vi "主程序-复材超声C扫缺陷分析评定软件.vi"() -> ()   [LabVIEW 2018]
doc: "使用该模板构建用户界面事件处理设计模式。将模板应用于对话框及其它用户界面。用户也可创建并执行VI可按照与用户界面事件相同方式处理的用户定义事件。"
uses:
  <vilib>/Utility/NIReport.llb/Report Type.ctl
  <vilib>/addons/_office/_exclsub.llb/font.ctl
  <vilib>/Utility/NIReport.llb/HTML Report Image Alignment.ctl
  <vilib>/Utility/NIReport.llb/Append Report Text (str wrap).vi
  <vilib>/Utility/NIReport.llb/Append Image to Report (path wrap).vi
  <vilib>/addons/_office/word.llb/Word Easy Table (str).vi
  <vilib>/Utility/NIReport.llb/NI_report.lvclass
  <vilib>/Utility/NIReport.llb/Word/NI_Word.lvclass
  <vilib>/addons/_office/NI_ReportGenerationToolkit.lvlib
  <vilib>/Utility/NIReport.llb/NI_ReportGenerationCore.lvlib
  <vilib>/vision/NI_Vision_Development_Module.lvlib
panel:
  out "报告模式":string
  in  "删除标注":bool caption="定量分析"
  out "输入的灰度阈值":dbl caption="值"
  out "反射图原始路径":path
  out "穿透图原始路径":path
  out "ROImask":T1(plugin-control)
  out "模式选择":u16(ring) items=["只读穿透图", "穿透图和反射图结合"]
  out "添加的路径":path
  out "连接的字符串 2":string
  out "临界面积百分比值":dbl
  out "临界Z值":i32
  out "标注后的图片路径":path
  out "弥散类检测结果合并":string[][](table)
  out "分层类检测结果合并":string[][](table)
  out "弥散类检测结果":string[][](table)
  out "分层类检测结果":string[][](table)
  out "部位信息":string[](array[string])=["", "34.500000", "32.500000", "1121", "34", "54.955926", "分层类", "不合格", ""]
  out "连接的字符串":string
  in  "完成标注":bool caption="定量分析"
  out "框数":dbl
  out "自定义字体":T2={"Desired Font (Application)"=enum."Application Font", "[User-specified Font]"={"Font Name"="", "Size"=12, "Strikeout?"=FALSE, "Italic?"=FALSE, "Underline?"=FALSE, "Outline?"=FALSE, "Shadow?"=FALSE, "Bold?"=FALSE, "Rotation Angle"=0.0}, "Horizontal Alignment"=0, "Vertical Alignment"=0} {"Horizontal Alignment" items=["Left", "Center", "Right"]; "Vertical Alignment" items=["Bottom", "Top", "Baseline"]}
  out "框组":T3(array[cluster])
  out "质量等级":string
  out "灰度阈值":dbl
  in  "stop":bool caption="停止"
  in  "导入图像":bool caption="导入图片"
  in  "开始标注":bool caption="定量分析"
  in  "查看评定结果":bool caption="辅助定性分析"
  in  "生成报告":bool caption="生成原始记录"
  in  "控件":enum32{"穿透图", "反射图"}(tab)
  out "穿透图":T1(plugin-control)
  out "反射图":T1(plugin-control)
  out "产品规格":cluster{"产品长度（周长）（mm）":dbl, "产品宽度（母线长）（mm）":dbl}
  out "图像分辨率":T4
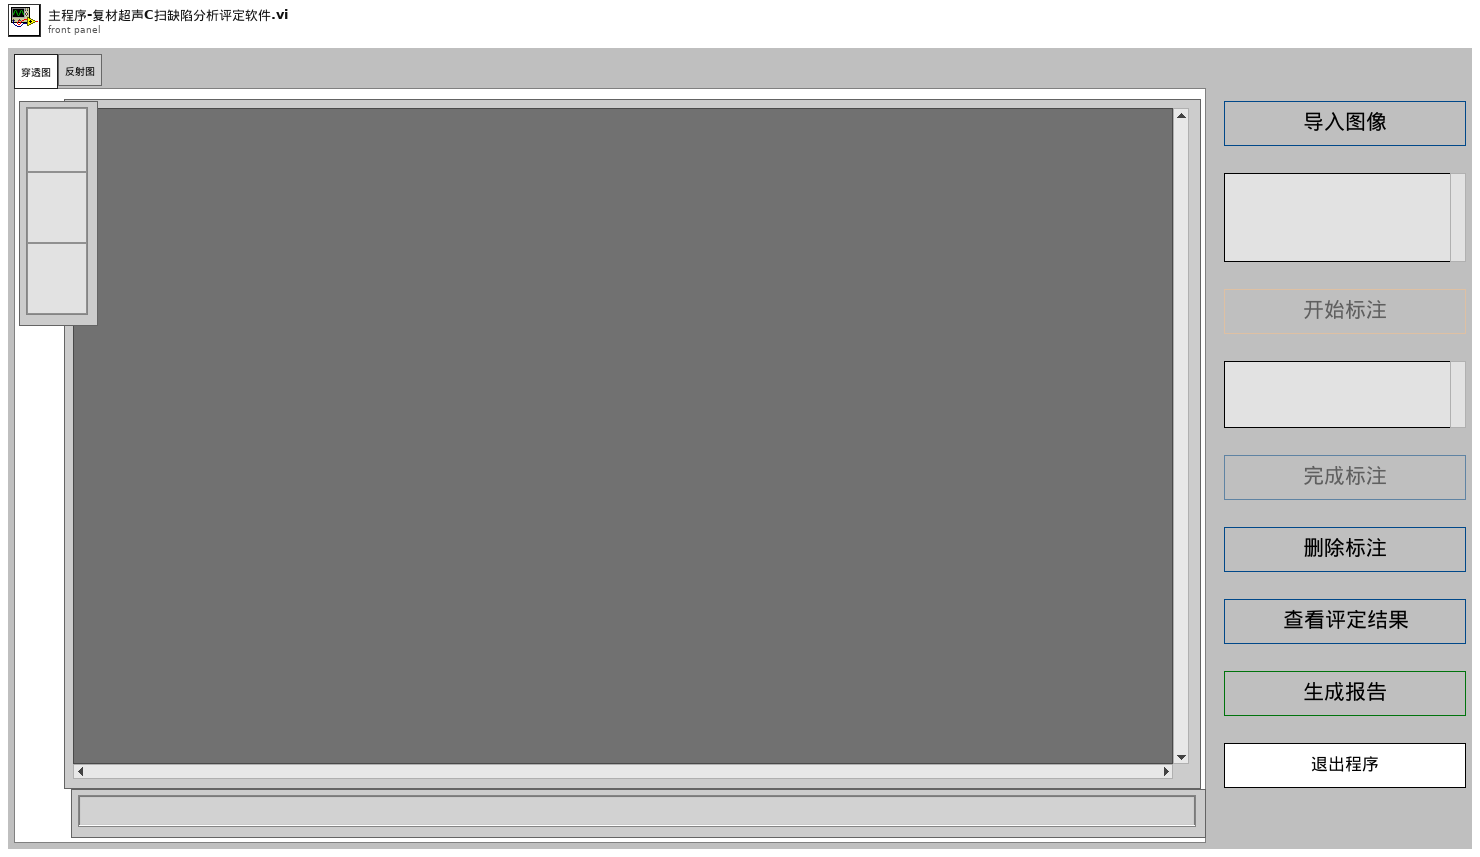
[diagram p1: front panel]
types:
  T1 = typedef "IMAQ Image.ctl" = refnum<image>
  T2 = cluster{"Desired Font (Application)":enum16{"User-specified Font", "Application Font", "System Font", "Dialog Font"}, "[User-specified Font]":cluster{"Font Name":string, "Size":i16, "Strikeout?":bool, "Italic?":bool, "Underline?":bool, "Outline?":bool, "Shadow?":bool, "Bold?":bool, "Rotation Angle":dbl}, "Horizontal Alignment":i16, "Vertical Alignment":i16}
  T3 = cluster{"Global Rectangle":i32[], "Contours":cluster{"Contour Type":u32, "ROI Type":u32, "Points":i32[]}[]}[]
  T4 = cluster{"图像X向分辨率（mm/像素）":dbl, "图像Y向分辨率（mm/像素）":dbl}
  T5 = enum8{"Enabled", "Disabled", "Disabled and Grayed Out"}
  T6 = cluster{"Global Rectangle":i32[], "Contours":cluster{"Contour Type":u32, "ROI Type":u32, "Points":i32[]}[]}
  T7 = cluster{"Zoom Tool":bool, "Selection Tool":bool, "Pan Tool":bool, "Point Tool":bool, "Line Tool":bool, "Rectangle Tool":bool, "Rotated Rectangle Tool":bool, "Polyline Tool":bool, "Polygon Tool":bool, "Freehand Tool":bool, "Closed Freehand Tool":bool, "Ellipse Tool":bool, "Annulus Tool":bool}
  T8 = enum16{"maximized", "minimized", "normal", "no change"}
  T9 = typedef "NI_ReportGenerationCore.lvlib/Report Type.ctl" = enum16{"HTML", "Word", "Excel"}
  T10 = cluster{"position (excel)":cluster{"row":i32, "column":i32}, "name (excel)":string, "bookmark (word)":string}
  T11 = typedef "NI_ReportGenerationCore.lvlib/HTML Report Image Alignment.ctl" = enum16{"(default)", "LEFT", "RIGHT", "TOP", "TEXTTOP", "MIDDLE", "ABSMIDDLE", "BASELINE", "BOTTOM", "ABSBOTTOM"}
  T12 = cluster{"position (Excel)":cluster{"row":i32, "column":i32}, "name (Excel)":string, "bookmark (Word)":string}
  T13 = typedef "NI_ReportGenerationToolkit.lvlib/font.ctl" = cluster{"font name":string, "font size":dbl, "bold":u16, "italic":u16, "underline":u16, "strike through":u16, "font color":u32}
  T14 = typedef "Image Type" = u32
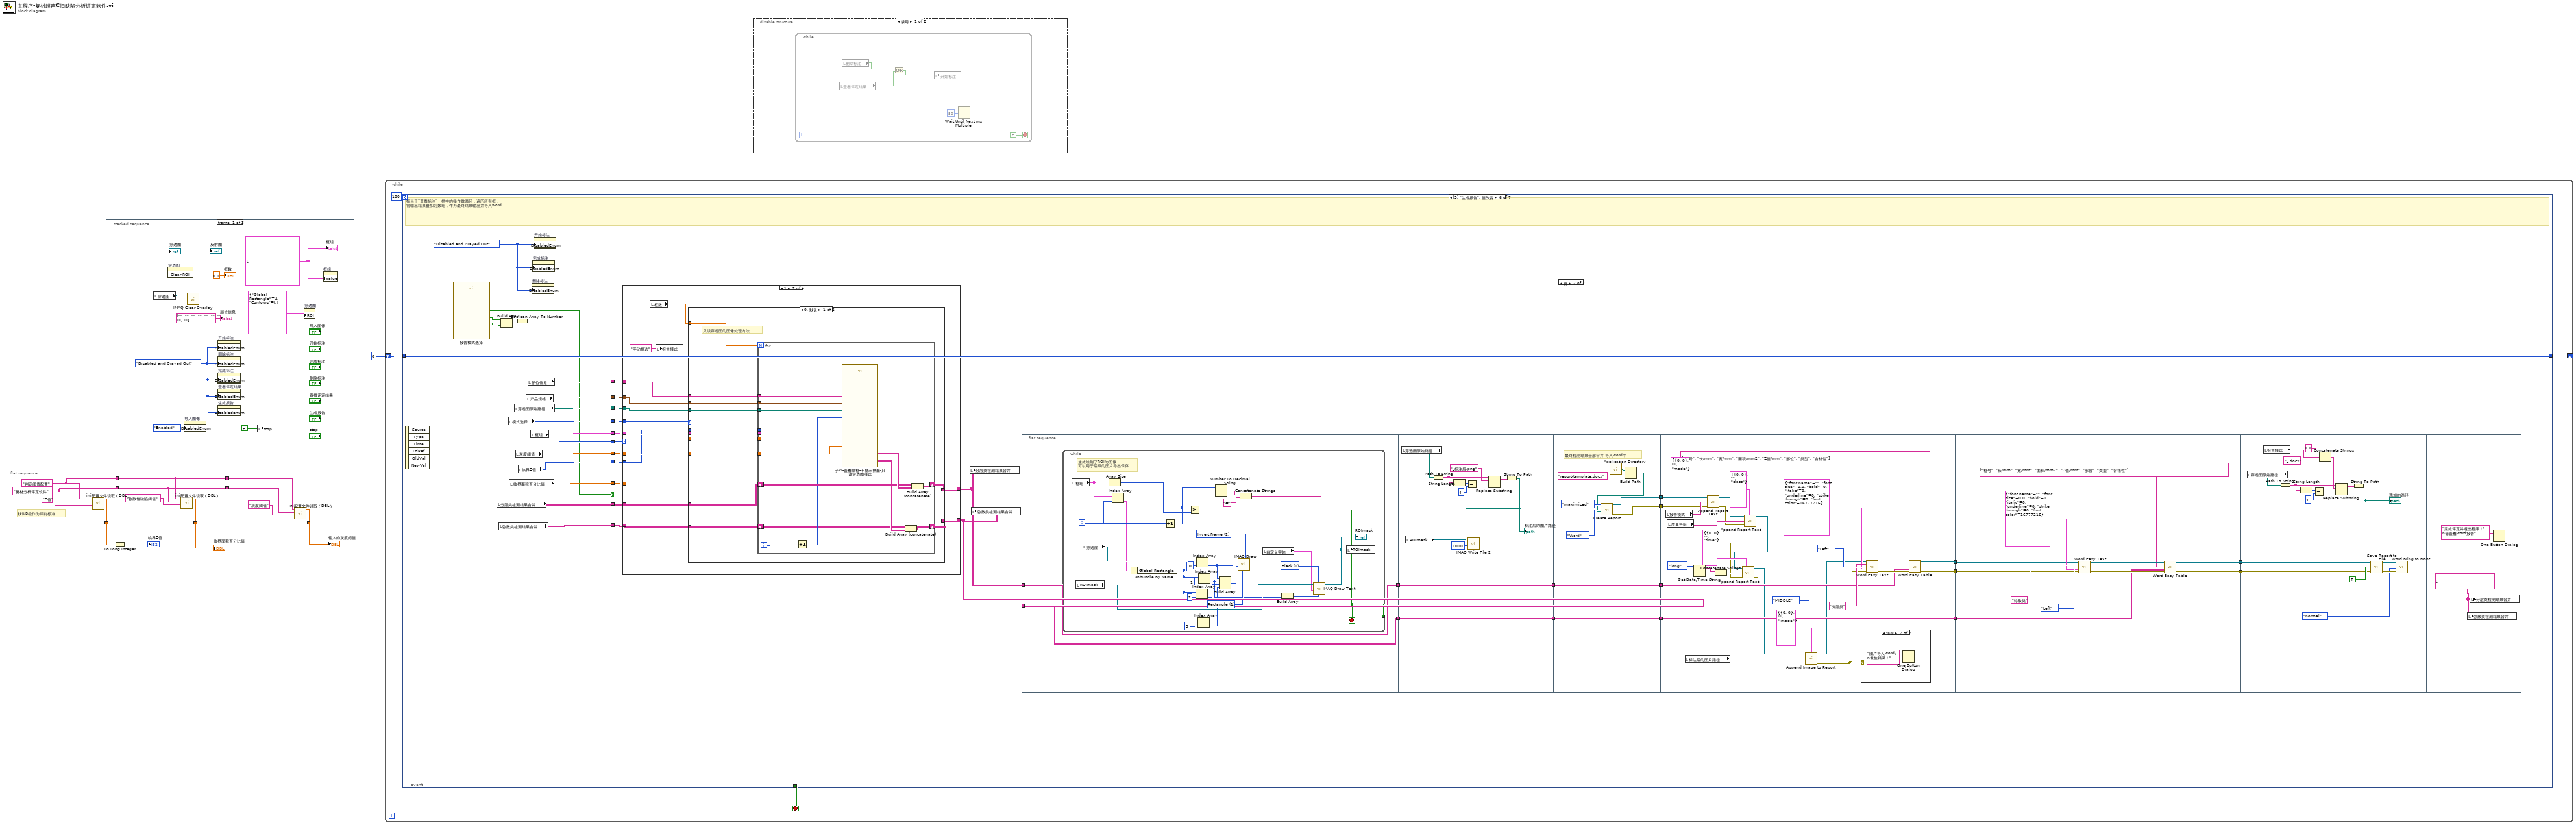
[diagram p0: block diagram]
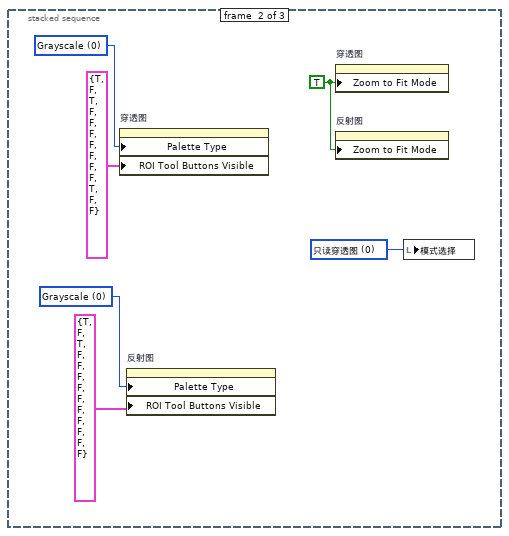
[diagram p2: hidden frame]
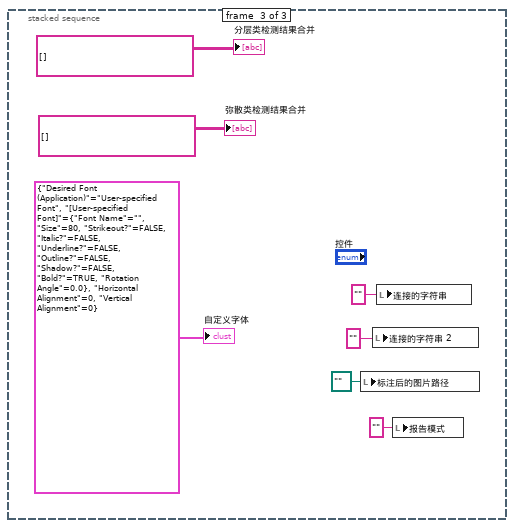
[diagram p3: hidden frame]
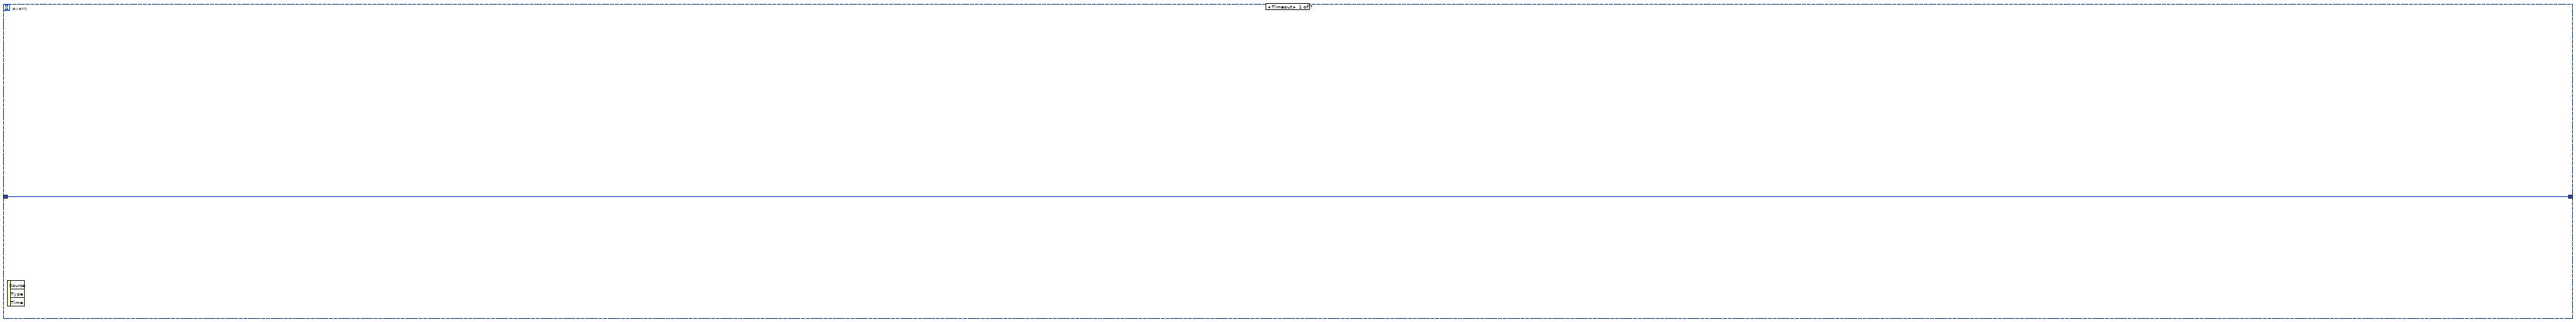
[diagram p5: hidden frame]
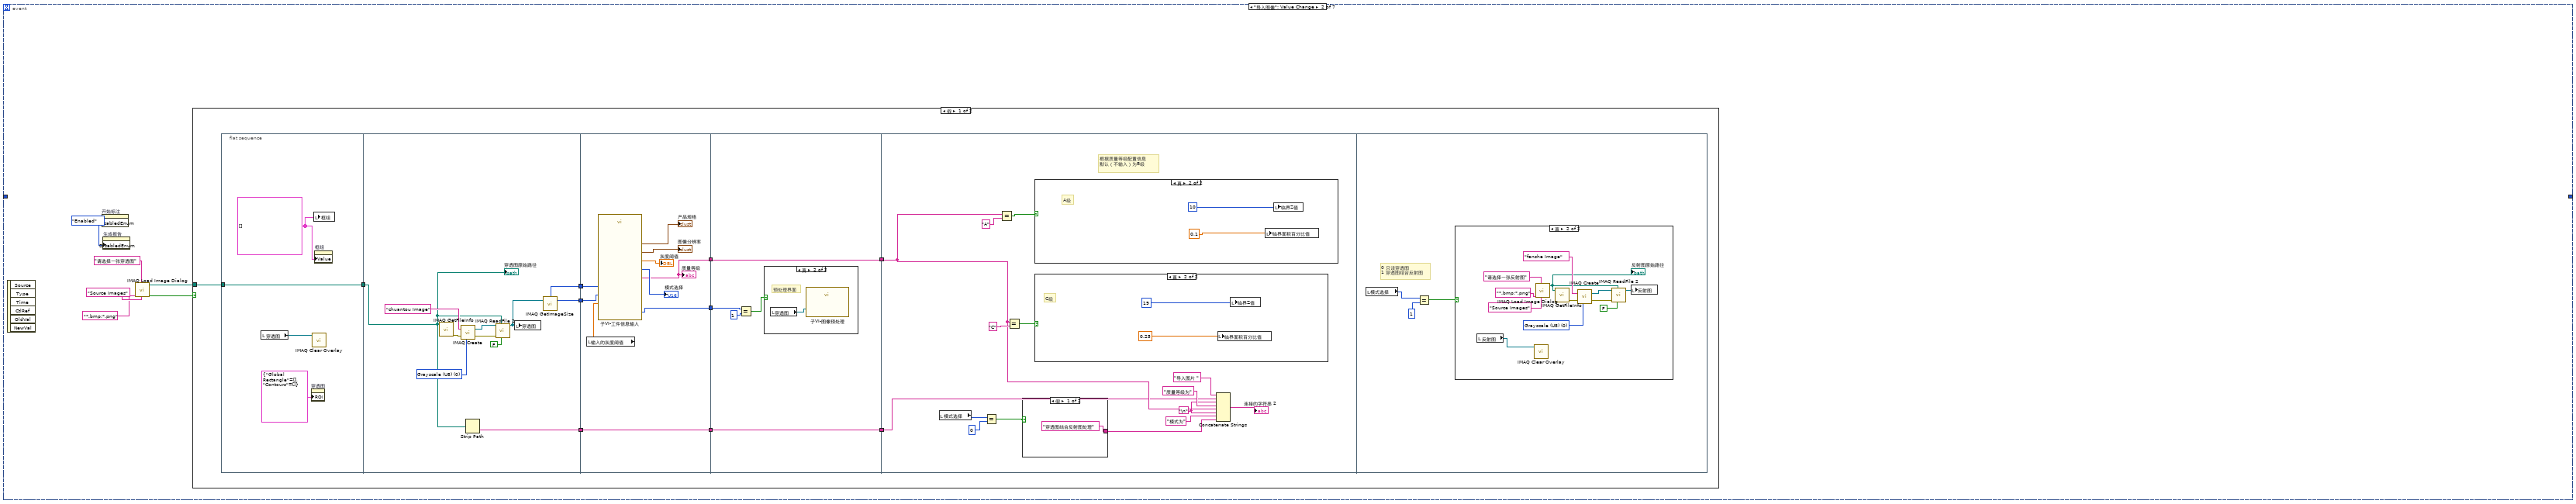
[diagram p6: hidden frame]
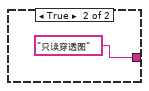
[diagram p8: hidden frame]
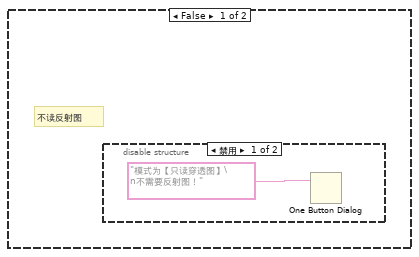
[diagram p11: hidden frame]
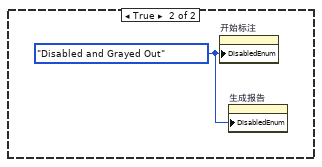
[diagram p13: hidden frame]
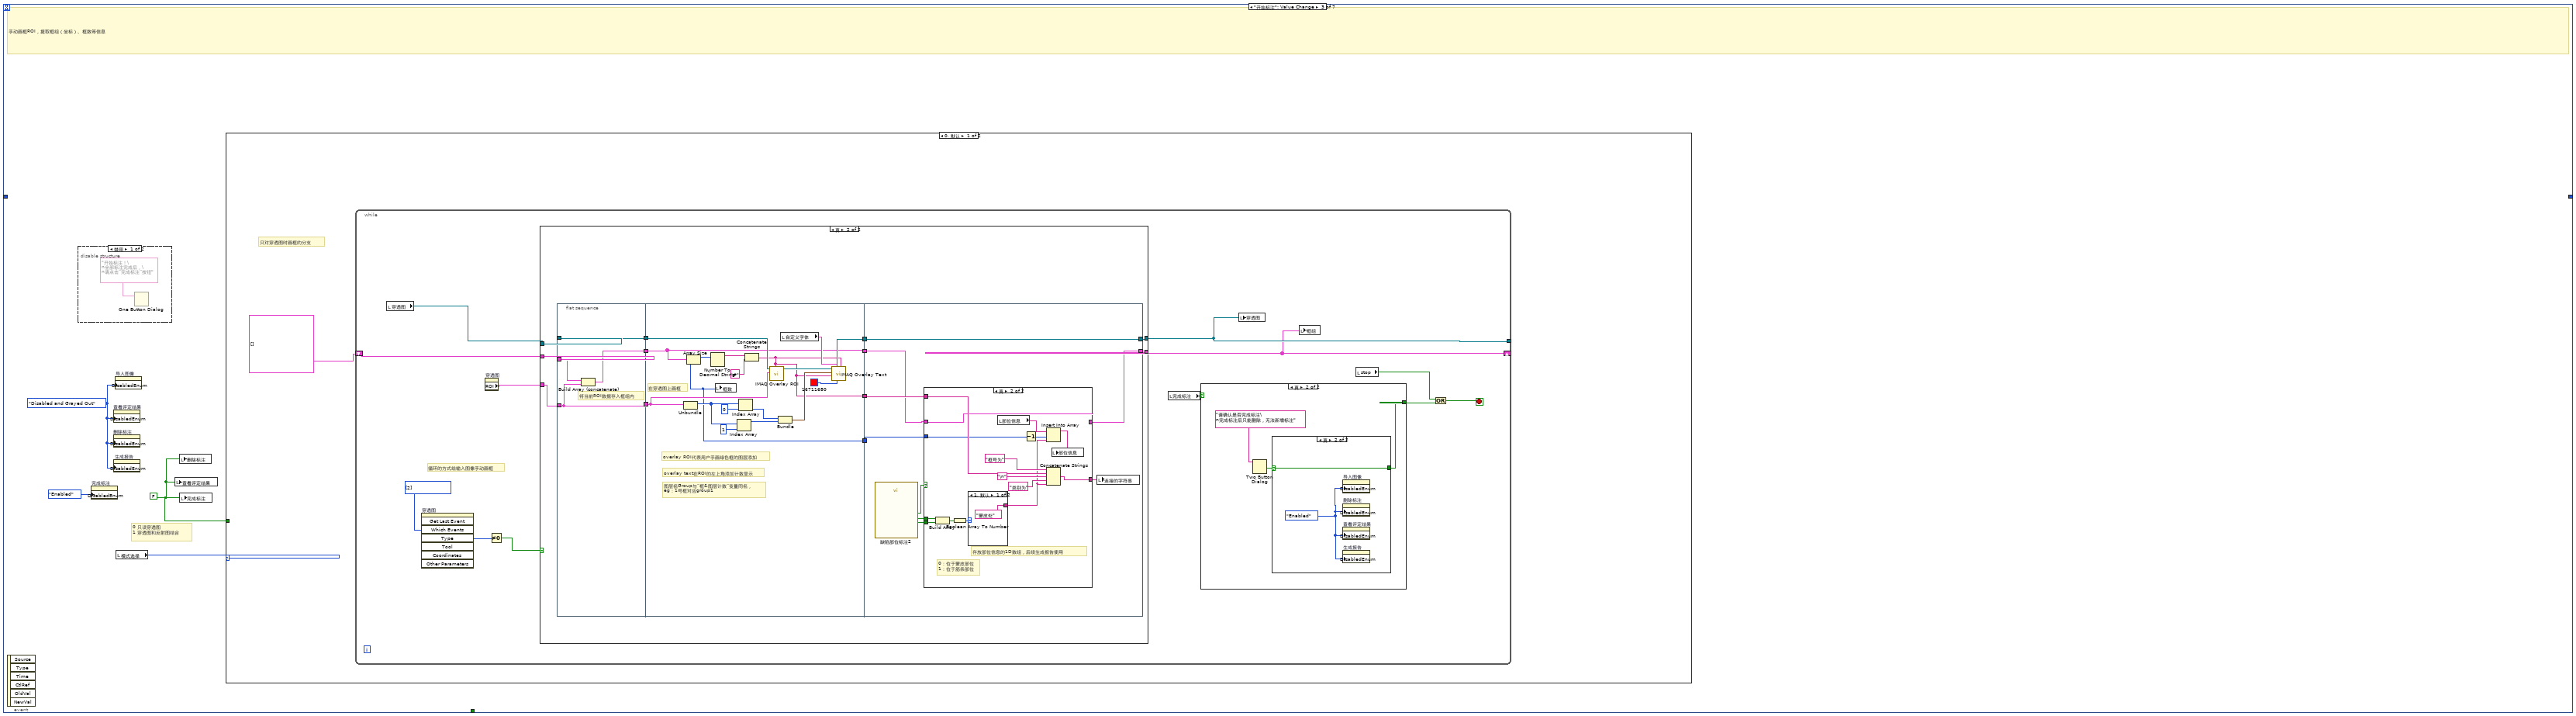
[diagram p14: hidden frame]
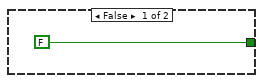
[diagram p16: hidden frame]
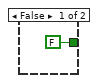
[diagram p17: hidden frame]
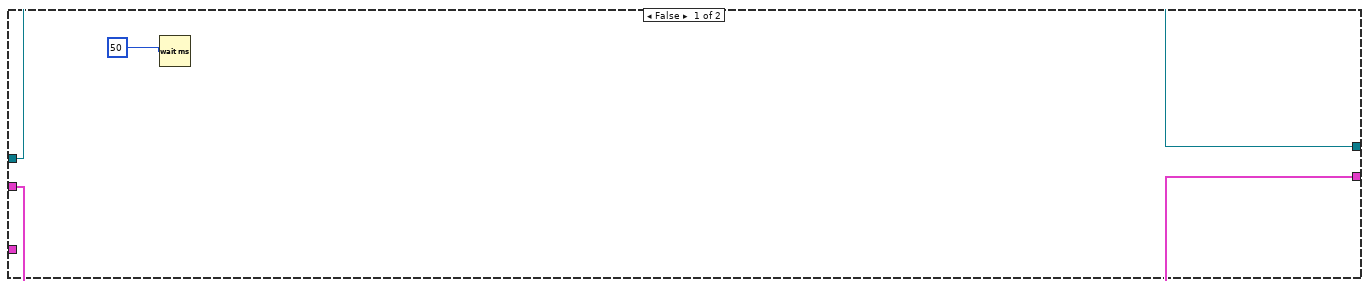
[diagram p18: hidden frame]
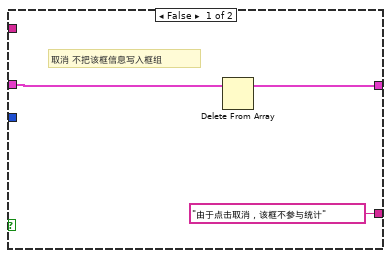
[diagram p19: hidden frame]
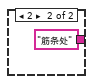
[diagram p20: hidden frame]
diagram:
  n1 = flat-sequence {
    tunnel: [w12] -> w8
    tunnel: [w11] -> w7
    tunnel: [w10] -> w2
    tunnel: w8 -> [w15]
    tunnel: w7 -> [w16]
    tunnel: [w16] -> w6
    tunnel: [w15] -> w5
    tunnel: [w14] -> w3
    tunnel: w6 -> [w20]
    tunnel: w5 -> [w19]
    tunnel: [w18] -> w4
    frame #0 {
      w11 = "复材分析评定软件" ("section")
      w12 = "判定阈值配置" ("文件名称")
      # "默认B级作为评判标准"
      n2 = call "ini配置文件读取（DBL）.vi"("key"="Z值", "section"=w11, "文件名称"=w12) -> ("value"=w10:dbl)  [unwired: 8 in]
    }
    frame #1 {
      n3 = call "ini配置文件读取（DBL）.vi"("key"="弥散性缺陷阈值", "section"=w16, "文件名称"=w15) -> ("value"=w14:dbl)  [unwired: 8 in]
    }
    frame #2 {
      n4 = call "ini配置文件读取（DBL）.vi"("key"="灰度阈值", "section"=w20, "文件名称"=w19) -> ("value"=w18:dbl)  [unwired: 8 in]
    }
  }
  n5 = stacked-sequence {
    frame #0 {
      w27 = T3 [] ("框组")
      w23 = T5."Disabled and Grayed Out" ("禁用")
      n6 = local read "穿透图"() -> (w25:T1)
      n7 = invoke on="穿透图" class="ImageControl" method="Clear ROI"() -> ()  [unwired: 3 in, 3 out]
      n8 = property on="导入图像" class="Bool"("DisabledEnum"=T5."Enabled" ("禁用")) -> ()  [unwired: 2 in, 2 out]
      n9 = call "IMAQ Clear Overlay"("Image"=w25) -> ()  [unwired: 9 in, 2 out]
      n10 = property on="开始标注" class="Bool"("DisabledEnum"=w23) -> ()  [unwired: 2 in, 2 out]
      n11 = property on="删除标注" class="Bool (严格)"("DisabledEnum"=w23) -> ()  [unwired: 2 in, 2 out]
      n12 = property on="完成标注" class="Bool (严格)"("DisabledEnum"=w23) -> ()  [unwired: 2 in, 2 out]
      n13 = property on="查看评定结果" class="Bool (严格)"("DisabledEnum"=w23) -> ()  [unwired: 2 in, 2 out]
      n14 = property on="生成报告" class="Bool"("DisabledEnum"=w23) -> ()  [unwired: 2 in, 2 out]
      n15 = local write "stop"(FALSE ("stop")) -> ()
      n16 = property on="穿透图" class="ImageControl"("ROI"=T6 {"Global Rectangle"=[], "Contours"=[]}) -> ()  [unwired: 2 in, 2 out]
      n17 = property on="框组" class="Arr (严格)"("Value"=w27) -> ()  [unwired: 2 in, 2 out]
      "部位信息" <- string[] ["", "", "", "", "", "", "", "", ""] ("部位信息")
      "框组" <- w27
      "框数" <- 0.0 ("框数")
    }
    frame #1 {
      w30 = u16 0 items=["只读穿透图", "穿透图和反射图结合"] ("模式选择")
      w32 = u32 0 items=["Grayscale", "Binary", "Gradient", "Rainbow", "Temperature", "User Defined", "Binary 16 Bit", "Gradient 16 Bit", "Rainbow 16 Bit", "Temperature 16 Bit", "User Defined 16 Bit"] ("Palette:Palette Type")
      w33 = TRUE ("Zoom to Fit Mode")
      w35 = u32 0 items=["Grayscale", "Binary", "Gradient", "Rainbow", "Temperature", "User Defined", "Binary 16 Bit", "Gradient 16 Bit", "Rainbow 16 Bit", "Temperature 16 Bit", "User Defined 16 Bit"] ("Palette:Palette Type")
      n18 = property on="穿透图" class="ImageControl"("Palette Type"=w35, "ROI Tool Buttons Visible"=T7 {"Zoom Tool"=TRUE, "Selection Tool"=FALSE, "Pan Tool"=TRUE, "Point Tool"=FALSE, "Line Tool"=FALSE, "Rectangle Tool"=FALSE, "Rotated Rectangle Tool"=FALSE, "Polyline Tool"=FALSE, "Polygon Tool"=FALSE, "Freehand Tool"=FALSE, "Closed Freehand Tool"=TRUE, "Ellipse Tool"=FALSE, "Annulus Tool"=FALSE} ("ROI Tool Buttons Visible:All Elements")) -> ()  [unwired: 2 in, 2 out]
      n19 = property on="反射图" class="ImageControl"("Palette Type"=w32, "ROI Tool Buttons Visible"=T7 {"Zoom Tool"=TRUE, "Selection Tool"=FALSE, "Pan Tool"=TRUE, "Point Tool"=FALSE, "Line Tool"=FALSE, "Rectangle Tool"=FALSE, "Rotated Rectangle Tool"=FALSE, "Polyline Tool"=FALSE, "Polygon Tool"=FALSE, "Freehand Tool"=FALSE, "Closed Freehand Tool"=FALSE, "Ellipse Tool"=FALSE, "Annulus Tool"=FALSE} ("ROI Tool Buttons Visible:All Elements")) -> ()  [unwired: 2 in, 2 out]
      n20 = property on="穿透图" class="ImageControl"("Zoom to Fit Mode"=w33) -> ()  [unwired: 2 in, 2 out]
      n21 = property on="反射图" class="ImageControl"("Zoom to Fit Mode"=w33) -> ()  [unwired: 2 in, 2 out]
      n22 = local write "模式选择"(w30) -> ()
    }
    frame #2 {
      n23 = local write "标注后的图片路径"(path "" ("标注后的图片路径")) -> ()
      n24 = local write "连接的字符串 2"("" ("连接的字符串 2")) -> ()
      n25 = local write "连接的字符串"("" ("连接的字符串")) -> ()
      n26 = local write "报告模式"("" ("报告模式")) -> ()
      "自定义字体" <- T2 {"Desired Font (Application)"=enum."User-specified Font", "[User-specified Font]"={"Font Name"="", "Size"=80, "Strikeout?"=FALSE, "Italic?"=FALSE, "Underline?"=FALSE, "Outline?"=FALSE, "Shadow?"=FALSE, "Bold?"=TRUE, "Rotation Angle"=0.0}, "Horizontal Alignment"=0, "Vertical Alignment"=0} ("Font, Size & Style")
      "分层类检测结果合并" <- string[][] [] ("弥散类检测结果合并")
      "弥散类检测结果合并" <- string[][] [] ("弥散类检测结果合并")
    }
  }
  n27 = To Long Integer(number=w2) -> (32bit integer=→"临界Z值":i32)
  n28 = while {
    shift-right: [w43] -> _
    shift-left: 0 -> [w44]
    stop <- w46 stop-if-true
    n29 = event shown="[5] \"生成报告\": 值改变" {
      selector: _ -> [_ _ _ _ _ _ _]
      dyn-events: _ -> [_ _ _ _ _ _ _]
      timeout: 100 -> [_ _ _ _ _ _ _]
      tunnel: [_ _ _ _ _ _ w737] -> w46
      tunnel: w44 -> [w47 _ _ _ _ w401 _]
      tunnel: [w47 _ _ _ _ w401 0] -> w43
      event Timeout {
        n30 = event-data() -> ()  [unwired: 1 in, 3 out]
      }
      event "导入图像": Value Change {
        w48 = T5."Enabled" ("禁用")
        n31 = event-data() -> ()  [unwired: 1 in, 6 out]
        n32 = property on="开始标注" class="Bool"("DisabledEnum"=w48) -> ()  [unwired: 2 in, 2 out]
        n33 = property on="生成报告" class="Bool"("DisabledEnum"=w48) -> ()  [unwired: 2 in, 2 out]
        n34 = call "IMAQ Load Image Dialog"("Pattern Label"="Source Images", "Prompt"="请选择一张穿透图" ("prompt"), "Pattern"="*.bmp;*.png") -> ("Cancelled?"=w50:bool, "Path"=w49:path)  [unwired: 6 in, 1 out]
        n35 = case shown="假" w50 {
          tunnel: w49 -> [w60 _]
          frame False {
            n36 = flat-sequence {
              tunnel: w60 -> [w64]
              tunnel: [w64] -> w59
              tunnel: w59 -> [w69]
              tunnel: [w71] -> w58
              tunnel: [w70] -> w57
              tunnel: [w68] -> w56
              tunnel: [w84] -> w63
              tunnel: [w82] -> w62
              tunnel: w58 -> [w81]
              tunnel: w57 -> [w80]
              tunnel: w56 -> [w79]
              tunnel: [w79] -> w55
              tunnel: w63 -> [w93]
              tunnel: [w93] -> w61
              tunnel: w62 -> [w91]
              tunnel: w55 -> [w89]
              tunnel: [w89] -> w54
              tunnel: w61 -> [w102]
              tunnel: w54 -> [w95]
              frame #0 {
                w65 = T3 [] ("框组")
                n37 = local read "穿透图"() -> (w67:T1)
                n38 = property on="穿透图" class="ImageControl"("ROI"=T6 {"Global Rectangle"=[], "Contours"=[]}) -> ()  [unwired: 2 in, 2 out]
                n39 = call "IMAQ Clear Overlay"("Image"=w67) -> ()  [unwired: 9 in, 2 out]
                n40 = local write "框组"(w65) -> ()
                n41 = property on="框组" class="Arr (严格)"("Value"=w65) -> ()  [unwired: 2 in, 2 out]
              }
              frame #1 {
                w73 = T14 0 items=["Grayscale (U8)", "Grayscale (I16)", "Grayscale (SGL)", "Complex (CSG)", "RGB (U32)", "HSL (U32)", "RGB (U64)", "Grayscale (U16)"] ("Image Type")
                n42 = call "IMAQ GetFileInfo"("File Path"=w69) -> ("error out"=w76:errorcluster)  [unwired: 4 in, 6 out]
                n43 = call "IMAQ Create"("Image Name"="chuantou Image", "Image Type"=w73, "error in (no error)"=w76) -> ("New Image"=w77:T1, "error out"=w78:errorcluster)  [unwired: 2 in]
                n44 = Strip Path(path=w69) -> (name=w68:string)  [unwired: 1 out]
                n45 = call "IMAQ ReadFile 2"("Use File Path Image Type"=FALSE, "File Path"=w69, "error in (no error)"=w78, "Image"=w77) -> ("Image Out"=w75:T1)  [unwired: 3 in, 4 out]
                n46 = local write "穿透图"(w75) -> ()
                n47 = call "IMAQ GetImageSize"("Image"=w75) -> ("Y Resolution"=w70:i32, "X Resolution"=w71:i32)  [unwired: 3 in, 1 out]
                "穿透图原始路径" <- w69
              }
              frame #2 {
                n48 = local read "输入的灰度阈值"() -> (w83:dbl)
                n49 = call "子VI-工件信息输入.vi"("Y Resolution"=w80, "X Resolution"=w81, "输入的灰度阈值"=w83) -> ("质量等级"=w84:string, "模式选择"=→"模式选择":u16, "灰度阈值"=→"灰度阈值":dbl, "产品规格"=→"产品规格":cluster{"产品长度（周长）（mm）":dbl, "产品宽度（母线长）（mm）":dbl}, "是否需要预处理"=w82:u16, "图像分辨率"=→"图像分辨率":T4)  [unwired: 3 in]
                "质量等级" <- w84
              }
              frame #3 {
                n50 = Equal?(x=w91, y=u16 1) -> (x = y?=w90:bool)
                n51 = case shown="真" w90 {
                  frame False {
                  }
                  frame True {
                    # "预处理界面"
                    n52 = local read "穿透图"() -> (w94:T1)
                    n53 = call "子VI-图像预处理.vi"("穿透图"=w94) -> ()  [unwired: 11 in]
                  }
                }
              }
              frame #4 {
                w97 = "\n"
                # "根据质量等级配置信息\n默认（不输入）为B级"
                n54 = local read "模式选择"() -> (w100:u16)
                n55 = Equal?(x=w100, y=u16 0) -> (x = y?=w99:bool)
                n56 = Equal?(x=w102, y="A") -> (x = y?=w105:bool)
                n57 = Equal?(x=w102, y="C") -> (x = y?=w106:bool)
                n58 = case shown="假" w99 {
                  tunnel: ["穿透图结合反射图处理" ("字符串") "只读穿透图" ("字符串")] -> w98
                  frame False {
                  }
                  frame True {
                  }
                }
                n59 = case shown="真" w105 {
                  frame False {
                  }
                  frame True {
                    # "A级"
                    n60 = local write "临界面积百分比值"(0.1 ("临界面积百分比值")) -> ()
                    n61 = local write "临界Z值"(10 ("临界Z值")) -> ()
                  }
                }
                n62 = case shown="真" w106 {
                  frame False {
                  }
                  frame True {
                    # "C级"
                    n63 = local write "临界面积百分比值"(0.25 ("临界面积百分比值")) -> ()
                    n64 = local write "临界Z值"(19 ("临界Z值")) -> ()
                  }
                }
                n65 = Concatenate Strings("导入图片 " ("字符串"), w95, w97, "质量等级为" ("字符串"), w102, w97, "模式为" ("字符串"), w98) -> (→"连接的字符串 2":string)
              }
              frame #5 {
                # "0 只读穿透图\n1 穿透图结合反射图"
                n66 = local read "模式选择"() -> (w117:u16)
                n67 = Equal?(x=w117, y=u16 1) -> (x = y?=w116:bool)
                n68 = case shown="真" w116 {
                  frame False {
                    # "不读反射图"
                    n69 = disable-structure shown="禁用" {
                      frame Disabled {
                        n70 = One Button Dialog(message="模式为【只读穿透图】\n不需要反射图！" ("消息")) -> ()  [unwired: 1 in, 1 out]
                      }
                      frame Enabled {
                      }
                    }
                  }
                  frame True {
                    w123 = T14 0 items=["Grayscale (U8)", "Grayscale (I16)", "Grayscale (SGL)", "Complex (CSG)", "RGB (U32)", "HSL (U32)", "RGB (U64)", "Grayscale (U16)"] ("Image Type")
                    n71 = local read "反射图"() -> (w120:T1)
                    n72 = call "IMAQ Clear Overlay"("Image"=w120) -> ()  [unwired: 9 in, 2 out]
                    n73 = call "IMAQ Load Image Dialog"("Pattern Label"="Source Images", "Prompt"="请选择一张反射图" ("prompt"), "Pattern"="*.bmp;*.png") -> ("Path"=w122:path)  [unwired: 6 in, 2 out]
                    "反射图原始路径" <- w122
                    n74 = call "IMAQ GetFileInfo"("File Path"=w122) -> ("error out"=w126:errorcluster)  [unwired: 4 in, 6 out]
                    n75 = call "IMAQ Create"("Image Name"="fanshe Image", "Image Type"=w123, "error in (no error)"=w126) -> ("New Image"=w127:T1, "error out"=w128:errorcluster)  [unwired: 2 in]
                    n76 = call "IMAQ ReadFile 2"("Use File Path Image Type"=FALSE, "File Path"=w122, "error in (no error)"=w128, "Image"=w127) -> ("Image Out"=w121:T1)  [unwired: 3 in, 4 out]
                    n77 = local write "反射图"(w121) -> ()
                  }
                }
              }
            }
          }
          frame True {
            w132 = T5."Disabled and Grayed Out" ("禁用")
            n78 = property on="开始标注" class="Bool"("DisabledEnum"=w132) -> ()  [unwired: 2 in, 2 out]
            n79 = property on="生成报告" class="Bool"("DisabledEnum"=w132) -> ()  [unwired: 2 in, 2 out]
          }
        }
      }
      event "开始标注": Value Change {
        w134 = T5."Disabled and Grayed Out" ("禁用")
        w135 = FALSE ("完成标注")
        # "0 只读穿透图\n1 穿透图和反射图结合"
        # "手动画框ROI，提取框组（坐标）、框数等信息"
        n80 = event-data() -> ()  [unwired: 1 in, 6 out]
        n81 = disable-structure shown="禁用" {
          frame Disabled {
            n82 = One Button Dialog(message="开始标注！\n全部标注完成后，\n请点击“完成标注”按钮" ("消息")) -> ()  [unwired: 1 in, 1 out]
          }
          frame Enabled {
          }
        }
        n83 = property on="完成标注" class="Bool (严格)"("DisabledEnum"=T5."Enabled" ("禁用")) -> ()  [unwired: 2 in, 2 out]
        n84 = property on="查看评定结果" class="Bool (严格)"("DisabledEnum"=w134) -> ()  [unwired: 2 in, 2 out]
        n85 = property on="删除标注" class="Bool (严格)"("DisabledEnum"=w134) -> ()  [unwired: 2 in, 2 out]
        n86 = property on="生成报告" class="Bool"("DisabledEnum"=w134) -> ()  [unwired: 2 in, 2 out]
        n87 = property on="导入图像" class="Bool"("DisabledEnum"=w134) -> ()  [unwired: 2 in, 2 out]
        n88 = local read "模式选择"() -> (w136:u16)
        n89 = local write "查看评定结果"(w135) -> ()
        n90 = local write "删除标注"(w135) -> ()
        n91 = local write "完成标注"(w135) -> ()
        n92 = case shown="0, 默认" w136 {
          tunnel: w135 -> [_ _]
          frame 0, Default {
            # "只对穿透图时画框的分支"
            n93 = while {
              shift-right: [w140] -> _
              shift-left: T3 [] ("框组") -> [w150]
              tunnel: [w148] -> _
              stop <- w139 stop-if-true
              (unwired) "_" ("名称或相对路径")
              (unwired) ".docx" ("名称或相对路径")
              w146 = i32[] [2] items=["No Event"=0, "Click Event"=1, "Draw Event"=2, "Size Event"=4, "Scroll Event"=5, "Double Click Event"=8] ("Which Events")
              # "循环的方式给输入图像手动画框"
              n94 = local read "穿透图"() -> (w149:T1)
              n95 = invoke on="穿透图" class="ImageControl" method="Get Last Event"("Which Events"=w146) -> ("Type"=w142:i32)  [unwired: 7 in, 7 out]
              n96 = property on="穿透图" class="ImageControl"() -> ("ROI"=w144:T6)  [unwired: 2 in, 2 out]
              n97 = Not Equal To 0?(x=w142) -> (x != 0?=w141:bool)
              n98 = case shown="真" w141 {
                tunnel: w149 -> [w161 w173]
                tunnel: [w161 w172] -> w148
                tunnel: [w159 w170] -> w140
                tunnel: w150 -> [w159 w171]
                tunnel: w144 -> [_ w169]
                frame False {
                  n99 = Wait (ms)(milliseconds to wait=u32 50 ("毫秒倍数")) -> ()  [unwired: 1 out]
                  n100 = Wait (ms)(milliseconds to wait=u32 50) -> ()  [unwired: 1 out]
                }
                frame True {
                  n101 = flat-sequence {
                    tunnel: w173 -> [w174]
                    tunnel: [w174] -> w168
                    tunnel: w169 -> [w177]
                    tunnel: [w177] -> w167
                    tunnel: w171 -> [w176]
                    tunnel: [w175] -> w166
                    tunnel: w168 -> [w186]
                    tunnel: w167 -> [w185]
                    tunnel: w166 -> [w178]
                    tunnel: [w188] -> w165
                    tunnel: [w178] -> w164
                    tunnel: [w182] -> w163
                    tunnel: [w180] -> w162
                    tunnel: w165 -> [w203]
                    tunnel: w164 -> [w197]
                    tunnel: w163 -> [w200]
                    tunnel: w162 -> [w199]
                    tunnel: [w203] -> w172
                    tunnel: [w196] -> w170
                    frame #0 {
                      # "将当前ROI数据存入框组内"
                      n102 = Build Array (concatenate)(w176, w177) -> (w175:T3)
                    }
                    frame #1 {
                      # "在穿透图上画框"
                      # "图层名Group与“框&图层计数”变量同名，\neg：1号框对应group1"
                      # "overlay text在ROI的左上角添加计数显示"
                      # "overlay ROI代表用户手画绿色框的图层添加"
                      n103 = Unbundle(w185) -> ("Global Rectangle"=w193:i32[])  [unwired: 1 out]
                      n104 = Array Size(array=w178) -> (size(s)=w180:i32)
                      n105 = Number To Decimal String(number=w180) -> (decimal integer string=w181:string)  [unwired: 1 in]
                      n106 = local write "框数"(w180) -> ()
                      n107 = Index Array(array=w193, index=1 ("索引")) -> (element=w191:i32)
                      n108 = Index Array(array=w193, index=0 ("索引")) -> (element=w192:i32)
                      n109 = Concatenate Strings(w181, "#" ("字符串")) -> (w182:string)
                      n110 = call "IMAQ Overlay ROI"("Group"=w182, "ROI Descriptor"=w185, "Image"=w186) -> ("Image Out"=w194:T1)  [unwired: 7 in, 1 out]
                      n111 = Bundle(w192, w191) -> (w187:cluster{i32, i32})  [unwired: 1 in]
                      n112 = local read "自定义字体"() -> (w184:T2)
                      n113 = call "IMAQ Overlay Text"("Group"=w182, "Text Color (black)"=u32 16711680, "Font, Size & Style"=w184, "String"=w182, "Origin"=w187, "Image"=w194) -> ("Image Out"=w188:T1)  [unwired: 4 in, 1 out]
                    }
                    frame #2 {
                      n114 = call "缺陷部位标注2"() -> ("位于筋条处"=w202:bool, "位于蒙皮处"=w201:bool, "确定"=w198:bool)  [unwired: 16 in, 1 out]
                      n115 = case shown="真" w198 {
                        tunnel: w202 -> [_ w219]
                        tunnel: w201 -> [_ w218]
                        tunnel: w200 -> [_ w214]
                        tunnel: w199 -> [_ w211]
                        tunnel: w197 -> [w206 w208]
                        tunnel: [w205 w208] -> w196
                        tunnel: ["由于点击取消，该框不参与统计" w207] -> w195
                        frame False {
                          # "取消 不把该框信息写入框组"
                          n116 = Delete From Array(array=w206) -> (array with subset deleted=w205:T3)  [unwired: 2 in, 1 out]
                        }
                        frame True {
                          # "0：位于蒙皮部位\n1：位于筋条部位"
                          # "存放部位信息的1D数组，后续生成报告使用"
                          n117 = Build Array(w218, w219) -> (w220:bool[])
                          n118 = Boolean Array To Number(Boolean array=w220) -> (number=w221:u32)
                          n119 = case shown="1, 默认" w221 {
                            tunnel: ["蒙皮处" ("t") "筋条处" ("t")] -> w209
                            frame 1, Default {
                            }
                            frame 2 {
                            }
                          }
                          n120 = local read "部位信息"() -> (w213:string[])
                          n121 = Decrement(x=w211) -> (x-1=w210:i32)
                          n122 = Insert Into Array(array=w213, index=w210, new element=w209) -> (w212:string[])
                          n123 = Concatenate Strings("框号为" ("字符串"), w214, "\n", "类别为" ("字符串"), w209) -> (w207:string)
                          n124 = local write "部位信息"(w212) -> ()
                        }
                      }
                      n125 = local write "连接的字符串"(w195) -> ()
                    }
                  }
                }
              }
              n126 = local read "完成标注"() -> (w145:bool)
              n127 = case shown="真" w145 {
                tunnel: [FALSE ("T button?") w152] -> w143
                frame False {
                }
                frame True {
                  n128 = Two Button Dialog(message="请确认是否完成标注\n完成标注后只能删除，无法新增标注" ("消息")) -> (T button?=w153:bool)  [unwired: 2 in]
                  n129 = case shown="真" w153 {
                    selector: w153 -> [_ w157]
                    tunnel: [FALSE w157] -> w152
                    frame False {
                    }
                    frame True {
                      w156 = T5."Enabled" ("禁用")
                      n130 = property on="导入图像" class="Bool"("DisabledEnum"=w156) -> ()  [unwired: 2 in, 2 out]
                      n131 = property on="删除标注" class="Bool (严格)"("DisabledEnum"=w156) -> ()  [unwired: 2 in, 2 out]
                      n132 = property on="查看评定结果" class="Bool (严格)"("DisabledEnum"=w156) -> ()  [unwired: 2 in, 2 out]
                      n133 = property on="生成报告" class="Bool"("DisabledEnum"=w156) -> ()  [unwired: 2 in, 2 out]
                    }
                  }
                }
              }
              n134 = local write "穿透图"(w148) -> ()
              n135 = local write "框组"(w140) -> ()
              n136 = local read "stop"() -> (w147:bool)
              n137 = Or(x=w147, y=w143) -> (x .or. y?=w139:bool)
              n138 = call <vilib>:"Application Directory.vi"() -> ()  [unwired: 1 out]
            }
          }
          frame 1 {
            # "对穿透图和反射图同时画框的分支"
            n139 = while {
              shift-right: [w227] -> _
              shift-left: T3 [] ("框组") -> [w236]
              tunnel: [w234] -> _
              tunnel: [w233] -> _
              stop <- w226 stop-if-true
              (unwired) "_" ("名称或相对路径")
              (unwired) ".docx" ("名称或相对路径")
              w232 = i32[] [2] items=["No Event"=0, "Click Event"=1, "Draw Event"=2, "Size Event"=4, "Scroll Event"=5, "Double Click Event"=8] ("Which Events")
              # "循环的方式给输入图像手动画框"
              n140 = local read "反射图"() -> (w235:T1)
              n141 = local read "穿透图"() -> (w229:T1)
              n142 = invoke on="穿透图" class="ImageControl" method="Get Last Event"("Which Events"=w232) -> ("Type"=w231:i32)  [unwired: 7 in, 7 out]
              n143 = Not Equal To 0?(x=w231) -> (x != 0?=w237:bool)
              n144 = case shown="真" w237 {
                tunnel: w229 -> [w248 w264]
                tunnel: [w248 w249] -> w234
                tunnel: [w247 w259] -> w227
                tunnel: w236 -> [w247 w263]
                tunnel: w235 -> [w246 w262]
                tunnel: [w246 w261] -> w233
                frame False {
                  n145 = Wait (ms)(milliseconds to wait=u32 50 ("毫秒倍数")) -> ()  [unwired: 1 out]
                }
                frame True {
                  n146 = property on="穿透图" class="ImageControl"() -> ("ROI"=w260:T6)  [unwired: 2 in, 2 out]
                  n147 = flat-sequence {
                    tunnel: w264 -> [w267]
                    tunnel: [w267] -> w258
                    tunnel: w260 -> [w269]
                    tunnel: [w269] -> w257
                    tunnel: w263 -> [w268]
                    tunnel: w262 -> [w266]
                    tunnel: [w266] -> w256
                    tunnel: [w265] -> w255
                    tunnel: w258 -> [w278]
                    tunnel: w257 -> [w277]
                    tunnel: w256 -> [w283]
                    tunnel: w255 -> [w270]
                    tunnel: [w284] -> w254
                    tunnel: [w282] -> w253
                    tunnel: [w270] -> w252
                    tunnel: [w274] -> w251
                    tunnel: [w272] -> w250
                    tunnel: w254 -> [w293]
                    tunnel: w253 -> [w301]
                    tunnel: w252 -> [w295]
                    tunnel: w251 -> [w297]
                    tunnel: w250 -> [w296]
                    tunnel: [w301] -> w261
                    tunnel: [w294] -> w259
                    tunnel: [w293] -> w249
                    frame #0 {
                      # "将当前ROI数据存入框组内"
                      n148 = Build Array (concatenate)(w268, w269) -> (w265:T3)
                    }
                    frame #1 {
                      w280 = u32[] [15663114] ("Colors (Green)")
                      w276 = u32 16711776 ("Text Color (black)")
                      # "在反射图上对应位置画框"
                      # "在穿透图上画框"
                      # "图层名Group与“框&图层计数”变量同名，\neg：1号框对应group1"
                      # "overlay text在ROI的左上角添加计数显示"
                      # "overlay ROI代表用户手画绿色框的图层添加"
                      n149 = Array Size(array=w270) -> (size(s)=w272:i32)
                      n150 = Unbundle(w277) -> ("Global Rectangle"=w289:i32[])  [unwired: 1 out]
                      n151 = Number To Decimal String(number=w272) -> (decimal integer string=w273:string)  [unwired: 1 in]
                      n152 = local write "框数"(w272) -> ()
                      n153 = Concatenate Strings(w273, "#" ("字符串")) -> (w274:string)
                      n154 = Index Array(array=w289, index=1 ("索引")) -> (element=w287:i32)
                      n155 = Index Array(array=w289, index=0 ("索引")) -> (element=w288:i32)
                      n156 = local read "自定义字体"() -> (w275:T2)
                      n157 = call "IMAQ Overlay ROI"("Colors (Green)"=w280, "Group"=w274, "ROI Descriptor"=w277, "Image"=w278) -> ("Image Out"=w290:T1)  [unwired: 6 in, 1 out]
                      n158 = call "IMAQ Overlay ROI"("Colors (Green)"=w280, "Group"=w274, "ROI Descriptor"=w277, "Image"=w283) -> ("Image Out"=w281:T1)  [unwired: 6 in, 1 out]
                      n159 = Bundle(w288, w287) -> (w279:cluster{i32, i32})  [unwired: 1 in]
                      n160 = call "IMAQ Overlay Text"("Group"=w274, "Text Color (black)"=w276, "Font, Size & Style"=w275, "String"=w274, "Origin"=w279, "Image"=w281) -> ("Image Out"=w282:T1)  [unwired: 4 in, 1 out]
                      n161 = call "IMAQ Overlay Text"("Group"=w274, "Text Color (black)"=w276, "Font, Size & Style"=w275, "String"=w274, "Origin"=w279, "Image"=w290) -> ("Image Out"=w284:T1)  [unwired: 4 in, 1 out]
                    }
                    frame #2 {
                      # "0：位于蒙皮部位\n1：位于筋条部位"
                      n162 = call "缺陷部位标注"() -> ("位于筋条处"=w299:bool, "位于蒙皮处"=w298:bool, "确定"=w291:bool)  [unwired: 16 in, 1 out]
                      n163 = Build Array(w298, w299) -> (w300:bool[])
                      n164 = case shown="真" w291 {
                        tunnel: w300 -> [_ w316]
                        tunnel: w297 -> [_ w312]
                        tunnel: w296 -> [_ w309]
                        tunnel: w295 -> [w304 w306]
                        tunnel: [w303 w306] -> w294
                        tunnel: ["由于点击取消，该框不参与统计" w305] -> w292
                        frame False {
                          # "取消 不把该框信息写入框组"
                          n165 = Delete From Array(array=w304) -> (array with subset deleted=w303:T3)  [unwired: 2 in, 1 out]
                        }
                        frame True {
                          # "存放部位信息的1D数组，后续生成报告使用"
                          n166 = Boolean Array To Number(Boolean array=w316) -> (number=w317:u32)
                          n167 = local read "部位信息"() -> (w311:string[])
                          n168 = case shown="1, 默认" w317 {
                            tunnel: ["蒙皮处" ("t") "筋条处" ("t")] -> w307
                            frame 1, Default {
                            }
                            frame 2 {
                            }
                          }
                          n169 = Decrement(x=w309) -> (x-1=w308:i32)
                          n170 = Insert Into Array(array=w311, index=w308, new element=w307) -> (w310:string[])
                          n171 = Concatenate Strings("框号为" ("字符串"), w312, "\n", "类别为" ("字符串"), w307) -> (w305:string)
                          n172 = local write "部位信息"(w310) -> ()
                        }
                      }
                      "连接的字符串" <- w292
                    }
                  }
                }
              }
              n173 = local read "完成标注"() -> (w225:bool)
              n174 = case shown="真" w225 {
                tunnel: [FALSE ("T button?") w239] -> w228
                frame False {
                }
                frame True {
                  n175 = Two Button Dialog(message="请确认是否完成标注\n完成标注后只能删除，无法新增标注" ("消息")) -> (T button?=w240:bool)  [unwired: 2 in]
                  n176 = case shown="真" w240 {
                    selector: w240 -> [_ w244]
                    tunnel: [FALSE w244] -> w239
                    frame False {
                    }
                    frame True {
                      w243 = T5."Enabled" ("禁用")
                      n177 = property on="生成报告" class="Bool"("DisabledEnum"=w243) -> ()  [unwired: 2 in, 2 out]
                      n178 = property on="删除标注" class="Bool (严格)"("DisabledEnum"=w243) -> ()  [unwired: 2 in, 2 out]
                      n179 = property on="查看评定结果" class="Bool (严格)"("DisabledEnum"=w243) -> ()  [unwired: 2 in, 2 out]
                      n180 = property on="导入图像" class="Bool"("DisabledEnum"=w243) -> ()  [unwired: 2 in, 2 out]
                    }
                  }
                }
              }
              n181 = local write "框组"(w227) -> ()
              n182 = local write "穿透图"(w234) -> ()
              n183 = local write "反射图"(w233) -> ()
              n184 = local read "stop"() -> (w230:bool)
              n185 = Or(x=w230, y=w228) -> (x .or. y?=w226:bool)
              n186 = call <vilib>:"Application Directory.vi"() -> ()  [unwired: 1 out]
            }
          }
        }
      }
      event "删除标注": Value Change {
        w321 = T5."Disabled and Grayed Out" ("禁用")
        n187 = event-data() -> ()  [unwired: 1 in, 6 out]
        n188 = call "用户输入2"() -> ("框号"=w322:dbl, "确定"=w323:bool)  [unwired: 17 in, 1 out]
        n189 = property on="生成报告" class="Bool"("DisabledEnum"=T5."Enabled" ("禁用")) -> ()  [unwired: 2 in, 2 out]
        n190 = property on="完成标注" class="Bool (严格)"("DisabledEnum"=w321) -> ()  [unwired: 2 in, 2 out]
        n191 = property on="开始标注" class="Bool"("DisabledEnum"=w321) -> ()  [unwired: 2 in, 2 out]
        n192 = case shown="真" w323 {
          tunnel: w322 -> [_ w324]
          frame False {
            # "用户取消操作"
          }
          frame True {
            n193 = stacked-sequence {
              tunnel: w324 -> [_ w331 _]
              frame #0 {
                # "1. 删除所有框"
                n194 = local read "穿透图"() -> (w325:T1)
                n195 = call "IMAQ Clear Overlay"("Image"=w325) -> ()  [unwired: 9 in, 2 out]
              }
              frame #1 {
                # "2. 删除框组中指定元素"
                n196 = local read "部位信息"() -> (w328:string[])
                n197 = local read "框组"() -> (w330:T3)
                n198 = Decrement(x=w331) -> (x-1=w327:dbl)
                n199 = Delete From Array(array=w328, index=w327) -> (array with subset deleted=w326:string[])  [unwired: 1 in, 1 out]
                n200 = Delete From Array(array=w330, index=w327) -> (array with subset deleted=w329:T3)  [unwired: 1 in, 1 out]
                n201 = local write "框组"(w329) -> ()
                n202 = local write "部位信息"(w326) -> ()
              }
              frame #2 {
                # "3. 重画所有框"
                n203 = while {
                  i -> [w344]
                  stop <- w335 stop-if-true
                  n204 = local read "框组"() -> (w339:T3)
                  n205 = local read "穿透图"() -> (w343:T1)
                  n206 = Array Size(array=w339) -> (size(s)=w340:i32)
                  n207 = Index Array(array=w339, index=w344) -> (element=w334:T6)
                  n208 = Increment(x=w344) -> (x+1=w351:i32)
                  n209 = local write "框数"(w340) -> ()
                  n210 = Greater Or Equal?(x=w351, y=w340) -> (x >= y?=w335:bool)
                  n211 = call "IMAQ Overlay ROI"("ROI Descriptor"=w334, "Image"=w343) -> ("Image Out"=w349:T1)  [unwired: 8 in, 1 out]
                  n212 = Unbundle(w334) -> ("Global Rectangle"=w341:i32[])  [unwired: 1 out]
                  n213 = Number To Decimal String(number=w351) -> (decimal integer string=w336:string)  [unwired: 1 in]
                  n214 = Index Array(array=w341, index=0 ("索引")) -> (element=w346:i32)
                  n215 = Index Array(array=w341, index=1 ("索引")) -> (element=w347:i32)
                  n216 = local read "自定义字体"() -> (w333:T2)
                  n217 = Concatenate Strings(w336, "#" ("字符串")) -> (w332:string)
                  n218 = Bundle(w346, w347) -> (w337:cluster{i32, i32})  [unwired: 1 in]
                  n219 = call "IMAQ Overlay Text"("Text Color (black)"=u32 16711680, "Font, Size & Style"=w333, "String"=w332, "Origin"=w337, "Image"=w349) -> ("Image Out"=w342:T1)  [unwired: 5 in, 1 out]
                  n220 = local write "穿透图"(w342) -> ()
                }
              }
            }
          }
        }
      }
      event "查看评定结果": Value Change {
        w352 = T5."Disabled and Grayed Out" ("禁用")
        # "查看指定框的详细信息，包括灰度和面积阈值分割后的结果，提取到的长宽面积等信息"
        n221 = event-data() -> ()  [unwired: 1 in, 6 out]
        n222 = local read "模式选择"() -> (w362:u16)
        n223 = property on="完成标注" class="Bool (严格)"("DisabledEnum"=w352) -> ()  [unwired: 2 in, 2 out]
        n224 = property on="开始标注" class="Bool"("DisabledEnum"=w352) -> ()  [unwired: 2 in, 2 out]
        n225 = local read "临界面积百分比值"() -> (w356:dbl)
        n226 = local read "穿透图原始路径"() -> (w359:path)
        n227 = local read "临界Z值"() -> (w357:i32)
        n228 = local read "灰度阈值"() -> (w353:dbl)
        n229 = local read "部位信息"() -> (w361:string[])
        n230 = local read "产品规格"() -> (w360:cluster{"产品长度（周长）（mm）":dbl, "产品宽度（母线长）（mm）":dbl})
        n231 = local read "框组"() -> (w358:T3)
        n232 = case shown="0, 默认" w362 {
          tunnel: w361 -> [w372 w382]
          tunnel: w360 -> [w371 w381]
          tunnel: w359 -> [w370 w380]
          tunnel: w358 -> [w369 w379]
          tunnel: w357 -> [w368 w378]
          tunnel: w356 -> [w367 w377]
          tunnel: [w364 w376] -> w355
          tunnel: [w365 w375] -> w354
          tunnel: w353 -> [w366 w374]
          frame 0, Default {
            # "只读穿透图的图像处理方法"
            n233 = call "子VI-查看某框-只读穿透图模式.vi"("输入框号（默认值0为整张图）"=0.0 ("框号"), "框组"=w369, "临界Z值"=w368, "临界面积百分比值"=w367, "预先配置的灰度阈值"=w366, "穿透图原始路径"=w370, "部位信息"=w372, "产品规格"=w371) -> ("弥散类检测结果"=w364:string[][], "分层类检测结果"=w365:string[][])  [unwired: 10 in]
          }
          frame 1 {
            # "穿透图和反射图结合的图像处理方法"
            n234 = local read "反射图原始路径"() -> (w383:path)
            n235 = call "子VI-查看某框.vi"("输入框号（默认值0为整张图）"=0.0 ("框号"), "框组"=w379, "临界Z值"=w378, "反射图原始路径"=w383, "临界面积百分比值"=w377, "预先配置的灰度阈值"=w374, "穿透图原始路径"=w380, "部位信息"=w382, "产品规格"=w381) -> ("弥散类检测结果"=w376:string[][], "分层类检测结果"=w375:string[][])  [unwired: 9 in]
          }
        }
        "弥散类检测结果" <- w355
        "分层类检测结果" <- w354
      }
      event "生成报告": Value Change {
        w385 = T5."Disabled and Grayed Out" ("禁用")
        # "相当于“查看标注”一栏中的操作做循环，遍历所有框，\n将输出结果叠加为数组，作为最终结果输出并导入word"
        n236 = event-data() -> ()  [unwired: 1 in, 6 out]
        n237 = call "报告模式选择"() -> ("深度学习方法"=w384:bool, "自动检测结果"=w387:bool, "手动框选结果"=w388:bool, "确定"=w386:bool)  [unwired: 15 in, 1 out]
        n238 = local read "分层类检测结果合并"() -> (w393:string[][])
        n239 = local read "弥散类检测结果合并"() -> (w391:string[][])
        n240 = Build Array(w388, w387, w384) -> (w390:bool[])
        n241 = local read "模式选择"() -> (w400:u16)
        n242 = local read "临界面积百分比值"() -> (w394:dbl)
        n243 = local read "穿透图原始路径"() -> (w397:path)
        n244 = local read "灰度阈值"() -> (w392:dbl)
        n245 = Boolean Array To Number(Boolean array=w390) -> (number=w389:u32)
        n246 = local read "临界Z值"() -> (w395:i32)
        n247 = local read "产品规格"() -> (w398:cluster{"产品长度（周长）（mm）":dbl, "产品宽度（母线长）（mm）":dbl})
        n248 = local read "部位信息"() -> (w399:string[])
        n249 = local read "框组"() -> (w396:T3)
        n250 = property on="删除标注" class="Bool (严格)"("DisabledEnum"=w385) -> ()  [unwired: 2 in, 2 out]
        n251 = property on="完成标注" class="Bool (严格)"("DisabledEnum"=w385) -> ()  [unwired: 2 in, 2 out]
        n252 = property on="开始标注" class="Bool"("DisabledEnum"=w385) -> ()  [unwired: 2 in, 2 out]
        n253 = case shown="真" w386 {
          tunnel: w400 -> [_ w414]
          tunnel: w399 -> [_ w413]
          tunnel: w398 -> [_ w412]
          tunnel: w397 -> [_ w411]
          tunnel: w396 -> [_ w410]
          tunnel: w395 -> [_ w409]
          tunnel: w394 -> [_ w408]
          tunnel: w393 -> [_ w407]
          tunnel: w392 -> [_ w406]
          tunnel: w391 -> [_ w405]
          tunnel: w389 -> [_ w404]
          frame False {
          }
          frame True {
            n254 = case shown="1" w404 {
              tunnel: [w430 w499 w571 w612] -> w416
              tunnel: [w429 w498 w570 w611] -> w415
              tunnel: w414 -> [w435 w506 w576 _]
              tunnel: w413 -> [w433 w509 w579 _]
              tunnel: w412 -> [w432 w508 w578 w620]
              tunnel: w411 -> [w434 w507 w577 w619]
              tunnel: w410 -> [w436 w505 w575 _]
              tunnel: w409 -> [w438 w502 w574 w618]
              tunnel: w408 -> [w439 w503 w573 w617]
              tunnel: w407 -> [w441 w501 w569 w615]
              tunnel: w406 -> [w437 w504 w572 _]
              tunnel: w405 -> [w440 w500 w568 w613]
              frame 0, Default {
                # "默认手动框选结果"
                n255 = local read "框数"() -> (w431:dbl)
                n256 = case shown="0, 默认" w435 {
                  tunnel: [w453 w481] -> w430
                  tunnel: [w452 w480] -> w429
                  tunnel: w441 -> [w443 w479]
                  tunnel: w440 -> [w442 w478]
                  tunnel: w439 -> [w446 w477]
                  tunnel: w438 -> [w444 w476]
                  tunnel: w437 -> [w445 w475]
                  tunnel: w436 -> [w447 w474]
                  tunnel: w434 -> [w448 w473]
                  tunnel: w433 -> [w450 w472]
                  tunnel: w432 -> [w449 w471]
                  tunnel: w431 -> [w451 w470]
                  frame 0, Default {
                    # "只读穿透图的图像处理方法"
                    n257 = for {
                      N: w451 -> [_]
                      shift-right: [w467] -> w453
                      shift-left: w443 -> [w466]
                      shift-right: [w461] -> w452
                      shift-left: w442 -> [w462]
                      tunnel: w450 -> [w460]
                      tunnel: w449 -> [w459]
                      tunnel: w448 -> [w458]
                      tunnel: w447 -> [w457]
                      tunnel: w446 -> [w456]
                      tunnel: w445 -> [w455]
                      tunnel: w444 -> [w454]
                      i -> [w465]
                      n258 = Increment(x=w465) -> (x+1=w464:i32)
                      n259 = call "子VI-查看某框-不显示界面-只读穿透图模式.vi"("框号"=w464, "框组"=w457, "临界Z值"=w454, "临界面积百分比值"=w456, "预先配置的灰度阈值"=w455, "穿透图原始路径"=w458, "部位信息"=w460, "产品规格"=w459) -> ("弥散类检测结果"=w463:string[][], "分层类检测结果"=w468:string[][])  [unwired: 10 in]
                      n260 = Build Array (concatenate)(w462, w463) -> (w461:string[][])
                      n261 = Build Array (concatenate)(w466, w468) -> (w467:string[][])
                    }
                  }
                  frame 1 {
                    # "穿透图和反射图结合的图像处理方法"
                    n262 = local read "反射图原始路径"() -> (w469:path)
                    n263 = for {
                      N: w470 -> [_]
                      shift-right: [w493] -> w481
                      shift-left: w479 -> [w495]
                      shift-right: [w492] -> w480
                      shift-left: w478 -> [w490]
                      tunnel: w477 -> [w489]
                      tunnel: w476 -> [w488]
                      tunnel: w475 -> [w487]
                      tunnel: w474 -> [w486]
                      tunnel: w473 -> [w483]
                      tunnel: w472 -> [w485]
                      tunnel: w471 -> [w484]
                      tunnel: w469 -> [w482]
                      i -> [w497]
                      n264 = Increment(x=w497) -> (x+1=w496:i32)
                      n265 = call "子VI-查看某框-不显示界面.vi"("框号"=w496, "框组"=w486, "临界Z值"=w488, "反射图原始路径"=w482, "临界面积百分比值"=w489, "预先配置的灰度阈值"=w487, "穿透图原始路径"=w483, "部位信息"=w485, "产品规格"=w484) -> ("弥散类检测结果"=w491:string[][], "分层类检测结果"=w494:string[][])  [unwired: 9 in]
                      n266 = Build Array (concatenate)(w495, w494) -> (w493:string[][])
                      n267 = Build Array (concatenate)(w490, w491) -> (w492:string[][])
                    }
                  }
                }
                "报告模式" <- "手动框选"
              }
              frame 1 {
                n268 = local read "框数"() -> (w510:dbl)
                n269 = local write "报告模式"("手动框选") -> ()
                n270 = case shown="0, 默认" w506 {
                  tunnel: [w523 w551] -> w499
                  tunnel: [w522 w550] -> w498
                  tunnel: w510 -> [w521 w549]
                  tunnel: w509 -> [w520 w548]
                  tunnel: w508 -> [w519 w547]
                  tunnel: w507 -> [w518 w546]
                  tunnel: w505 -> [w517 w544]
                  tunnel: w504 -> [w516 w543]
                  tunnel: w503 -> [w515 w542]
                  tunnel: w502 -> [w514 w545]
                  tunnel: w501 -> [w513 w540]
                  tunnel: w500 -> [w512 w539]
                  frame 0, Default {
                    # "只读穿透图的图像处理方法"
                    n271 = for {
                      N: w521 -> [_]
                      shift-right: [w537] -> w523
                      shift-left: w513 -> [w536]
                      shift-right: [w531] -> w522
                      shift-left: w512 -> [w532]
                      tunnel: w520 -> [w530]
                      tunnel: w519 -> [w529]
                      tunnel: w518 -> [w528]
                      tunnel: w517 -> [w527]
                      tunnel: w516 -> [w526]
                      tunnel: w515 -> [w525]
                      tunnel: w514 -> [w524]
                      i -> [w535]
                      n272 = Increment(x=w535) -> (x+1=w534:i32)
                      n273 = call "子VI-查看某框-不显示界面-只读穿透图模式.vi"("框号"=w534, "框组"=w527, "临界Z值"=w524, "临界面积百分比值"=w525, "预先配置的灰度阈值"=w526, "穿透图原始路径"=w528, "部位信息"=w530, "产品规格"=w529) -> ("弥散类检测结果"=w533:string[][], "分层类检测结果"=w538:string[][])  [unwired: 10 in]
                      n274 = Build Array (concatenate)(w532, w533) -> (w531:string[][])
                      n275 = Build Array (concatenate)(w536, w538) -> (w537:string[][])
                    }
                  }
                  frame 1 {
                    # "穿透图和反射图结合的图像处理方法"
                    n276 = local read "反射图原始路径"() -> (w541:path)
                    n277 = for {
                      N: w549 -> [_]
                      shift-right: [w563] -> w551
                      shift-left: w540 -> [w565]
                      shift-right: [w562] -> w550
                      shift-left: w539 -> [w560]
                      tunnel: w548 -> [w559]
                      tunnel: w547 -> [w558]
                      tunnel: w546 -> [w557]
                      tunnel: w545 -> [w556]
                      tunnel: w544 -> [w555]
                      tunnel: w543 -> [w554]
                      tunnel: w542 -> [w553]
                      tunnel: w541 -> [w552]
                      i -> [w567]
                      n278 = Increment(x=w567) -> (x+1=w566:i32)
                      n279 = call "子VI-查看某框-不显示界面.vi"("框号"=w566, "框组"=w555, "临界Z值"=w556, "反射图原始路径"=w552, "临界面积百分比值"=w553, "预先配置的灰度阈值"=w554, "穿透图原始路径"=w557, "部位信息"=w559, "产品规格"=w558) -> ("弥散类检测结果"=w561:string[][], "分层类检测结果"=w564:string[][])  [unwired: 9 in]
                      n280 = Build Array (concatenate)(w565, w564) -> (w563:string[][])
                      n281 = Build Array (concatenate)(w560, w561) -> (w562:string[][])
                    }
                  }
                }
              }
              frame 2 {
                n282 = local write "报告模式"("自动检测") -> ()
                n283 = case shown="1" w576 {
                  tunnel: [w594 w609] -> w571
                  tunnel: [w593 w608] -> w570
                  tunnel: w579 -> [w589 w604]
                  tunnel: w578 -> [w588 w603]
                  tunnel: w577 -> [w587 w602]
                  tunnel: w575 -> [w586 w600]
                  tunnel: w574 -> [w585 w597]
                  tunnel: w573 -> [w584 w598]
                  tunnel: w572 -> [w583 w599]
                  tunnel: w569 -> [w582 w596]
                  tunnel: w568 -> [w581 w595]
                  frame 0, Default {
                    # "只读穿透图的图像处理方法"
                    n284 = call "子VI-查看某框-不显示界面-只读穿透图模式.vi"("框号"=0.0, "框组"=w586, "临界Z值"=w585, "临界面积百分比值"=w584, "预先配置的灰度阈值"=w583, "穿透图原始路径"=w587, "部位信息"=w589, "产品规格"=w588) -> ("弥散类检测结果"=w591:string[][], "分层类检测结果"=w592:string[][])  [unwired: 10 in]
                    n285 = Build Array (concatenate)(w581, w591) -> (w593:string[][])
                    n286 = Build Array (concatenate)(w582, w592) -> (w594:string[][])
                  }
                  frame 1 {
                    # "穿透图和反射图结合的图像处理方法"
                    n287 = local read "反射图原始路径"() -> (w601:path)
                    n288 = call "子VI-查看某框-不显示界面.vi"("框号"=0.0, "框组"=w600, "临界Z值"=w597, "反射图原始路径"=w601, "临界面积百分比值"=w598, "预先配置的灰度阈值"=w599, "穿透图原始路径"=w602, "部位信息"=w604, "产品规格"=w603) -> ("弥散类检测结果"=w606:string[][], "分层类检测结果"=w607:string[][])  [unwired: 9 in]
                    n289 = Build Array (concatenate)(w596, w607) -> (w609:string[][])
                    n290 = Build Array (concatenate)(w595, w606) -> (w608:string[][])
                  }
                }
              }
              frame 4 {
                # "深度学习方法自动检测demo"
                n291 = local write "报告模式"("深度学习自动检测" ("报告模式")) -> ()
                n292 = call "子VI-深度学习自动检测.vi"("穿透图原始路径"=w619, "产品规格"=w620, "临界面积百分比值"=w617, "临界Z值"=w618) -> ("弥散类检测结果"=w614:string[][], "分层类检测结果"=w616:string[][])  [unwired: 6 in]
                n293 = Build Array (concatenate)(w614, w613) -> (w611:string[][])
                n294 = Build Array (concatenate)(w616, w615) -> (w612:string[][])
              }
            }
            n295 = local write "分层类检测结果合并"(w416) -> ()
            n296 = local write "弥散类检测结果合并"(w415) -> ()
            n297 = flat-sequence {
              tunnel: w415 -> [w621]
              tunnel: w416 -> [w622]
              tunnel: [w622] -> w427
              tunnel: [w621] -> w426
              tunnel: w427 -> [w662]
              tunnel: [w662] -> w425
              tunnel: w426 -> [w661]
              tunnel: [w661] -> w424
              tunnel: w425 -> [w669]
              tunnel: w424 -> [w668]
              tunnel: [w669] -> w423
              tunnel: [w668] -> w422
              tunnel: [w664] -> w403
              tunnel: [w663] -> w402
              tunnel: [w697] -> w421
              tunnel: [w696] -> w420
              tunnel: w423 -> [w689]
              tunnel: w422 -> [w690]
              tunnel: [w690] -> w419
              tunnel: w403 -> [w679]
              tunnel: w402 -> [w678]
              tunnel: w421 -> [w709]
              tunnel: w420 -> [w708]
              tunnel: w419 -> [w707]
              tunnel: [w706] -> w418
              tunnel: [w705] -> w417
              tunnel: w418 -> [w728]
              tunnel: w417 -> [w727]
              frame #0 {
                n298 = while {
                  tunnel: [w639] -> _
                  i -> [w641]
                  stop <- w639 stop-if-true
                  w646 = 1 items=["White", "Black", "Inverted", "Black on White", "White on Black"] ("Color")
                  w648 = u16 2 items=["Frame", "Paint", "Invert Frame", "Invert Paint"] ("Draw Mode")
                  w643 = u16 1 items=["Line", "Rectangle", "Oval"] ("Shape to draw")
                  # "生成绘制了ROI的图像\n可以用于后续的图片导出保存"
                  n299 = local read "框组"() -> (w640:T3)
                  n300 = local read "ROImask"() -> (w636:T1)
                  n301 = local read "穿透图"() -> (w637:T1)
                  n302 = Array Size(array=w640) -> (size(s)=w649:i32)
                  n303 = Index Array(array=w640, index=w641) -> (element=w634:T6)
                  n304 = Unbundle By Name(w634) -> ("Global Rectangle"=w629:i32[])
                  n305 = Increment(x=w641) -> (x+1=w650:i32)
                  n306 = Greater Or Equal?(x=w650, y=w649) -> (x >= y?=w639:bool)
                  n307 = Index Array(array=w629, index=2 ("索引")) -> (element=w628:i32)
                  n308 = Index Array(array=w629, index=0 ("索引")) -> (element=w625:i32)
                  n309 = Index Array(array=w629, index=3 ("索引")) -> (element=w627:i32)
                  n310 = Index Array(array=w629, index=1 ("索引")) -> (element=w624:i32)
                  n311 = Number To Decimal String(number=w650) -> (decimal integer string=w644:string)  [unwired: 1 in]
                  n312 = Build Array(w625, w624, w628, w627) -> (w626:i32[])
                  n313 = call "IMAQ Draw"("Draw Mode"=w648, "Shape to draw"=w643, "Coordinates"=w626, "Image Src"=w637) -> ("Image Dst Out"=w647:T1)  [unwired: 6 in, 1 out]
                  n314 = Concatenate Strings(w644, "#" ("字符串")) -> (w642:string)
                  n315 = local read "自定义字体"() -> (w638:T2)
                  n316 = Build Array(w625, w624) -> (w623:i32[])
                  n317 = call "IMAQ Draw Text"("String"=w642, "Insertion Point"=w623, "Color"=w646, "Font, Size & Style"=w638, "Image Dst"=w636, "Image Src"=w647) -> ("Image Dst Out"=w635:T1)  [unwired: 2 in, 3 out]
                  "ROImask" <- w635
                  n318 = local write "ROImask"(w635) -> ()
                }
              }
              frame #1 {
                n319 = local read "穿透图原始路径"() -> (w660:path)
                n320 = local read "ROImask"() -> (w651:T1)
                n321 = Path To String(path=w660) -> (string=w657:string)
                n322 = String Length(string=w657) -> (length=w658:i32)
                n323 = Subtract(x=w658, y=4) -> (x-y=w659:i32)
                n324 = Replace Substring(3:w659, 4:"_标注后.png" ("字符串"), 5:w657) -> (1:w656:string)  [unwired: 1 in, 1 out]
                n325 = String To Path(string=w656) -> (path=w652:path)
                "标注后的图片路径" <- w652
                n326 = call-poly "IMAQ Write File 2"("Image Quality"=u32 1000, "File Path"=w652, "Image"=w651) -> ()  [unwired: 7 in, 2 out]
              }
              frame #2 {
                # "最终检测结果全部合并 导入word中"
                n327 = call <vilib>:"Application Directory.vi"() -> ("Application Directory"=w667:path)
                n328 = Build Path(base path=w667, name or relative path="report-template.docx") -> (appended path=w665:path)
                n329 = call <vilib>:"Create Report.vi"("window state (normal)"=T8."maximized", "report type"=Report_Type."Word", "template (empty)"=w665) -> ("report out"=w664:refnum<class "NI_report.lvclass">, "error out"=w663:errorcluster)  [unwired: 11 in]
              }
              frame #3 {
                n330 = local read "报告模式"() -> (w680:string)
                n331 = local read "质量等级"() -> (w676:string)
                n332 = local read "标注后的图片路径"() -> (w687:path)
                n333 = Get Date/Time String(date format (0)=enum16{"short", "long", "abbreviated"}."long" ("日期格式(0)")) -> (date string=w694:string, time string=w695:string)  [unwired: 2 in]
                n334 = call-poly <vilib>:"Append Report Text.vi"("report in"=w679, "MS Office parameters"=T10 {"position (excel)"={"row"=0, "column"=0}, "name (excel)"="", "bookmark (word)"="mode"}, "text"=w680, "error in (no error)"=w678) -> ("report out"=w675:refnum<class "NI_report.lvclass">, "error out"=w674:errorcluster)  [unwired: 8 in, 2 out]
                n335 = Concatenate Strings(w694, w695) -> (w693:string)
                n336 = call-poly <vilib>:"Append Report Text.vi"("report in"=w675, "MS Office parameters"=T10 {"position (excel)"={"row"=0, "column"=0}, "name (excel)"="", "bookmark (word)"="class"}, "text"=w676, "error in (no error)"=w674) -> ("report out"=w672:refnum<class "NI_report.lvclass">, "error out"=w673:errorcluster)  [unwired: 8 in, 2 out]
                n337 = call-poly <vilib>:"Append Report Text.vi"("report in"=w672, "MS Office parameters"=T10 {"position (excel)"={"row"=0, "column"=0}, "name (excel)"="", "bookmark (word)"="time"}, "text"=w693, "error in (no error)"=w673) -> ("report out"=w686:refnum<class "NI_report.lvclass">, "error out"=w684:errorcluster)  [unwired: 8 in, 2 out]
                n338 = call-poly <vilib>:"Append Image to Report.vi"("report in"=w686, "alignment (default)"=HTML_Report_Image_Alignment."MIDDLE", "MS Office parameters"=T12 {"position (Excel)"={"row"=0, "column"=0}, "name (Excel)"="", "bookmark (Word)"="image"}, "path or URL of image"=w687, "error in (no error)"=w684) -> ("report out"=w683:refnum<class "NI_report.lvclass">, "error out"=w682:errorcluster)  [unwired: 7 in, 2 out]
                n339 = case shown="错误" w682 {
                  frame No Error {
                  }
                  frame Error {
                    n340 = One Button Dialog(message="图片导入word\n发生错误！" ("消息")) -> ()  [unwired: 1 in, 1 out]
                  }
                }
                n341 = call <vilib>:"Word Easy Text.vi"("report in"=w683, "text"="分层类", "alignment (left)"=enum16{"Left", "Centered", "Right", "Justify"}."Left", "font"=T13 {"font name"="", "font size"=0.0, "bold"=0, "italic"=0, "underline"=0, "strike through"=0, "font color"=16777216}, "error in (no error)"=w682) -> ("report out"=w699:refnum<class "NI_report.lvclass">, "error out"=w700:errorcluster)  [unwired: 8 in, 1 out]
                n342 = call-poly <vilib>:"Word Easy Table.vi"("report in"=w699, "column headers"=string[] ["框号", "长/mm", "宽/mm", "面积/mm2", "Z值/mm", "部位", "类型", "合格性"], "data"=w689, "error in (no error)"=w700) -> ("report out"=w697:refnum<class "NI_report.lvclass">, "error out"=w696:errorcluster)  [unwired: 9 in, 1 out]
              }
              frame #4 {
                n343 = call <vilib>:"Word Easy Text.vi"("report in"=w709, "text"="弥散类", "alignment (left)"=enum16{"Left", "Centered", "Right", "Justify"}."Left", "font"=T13 {"font name"="", "font size"=0.0, "bold"=0, "italic"=0, "underline"=0, "strike through"=0, "font color"=16777216}, "error in (no error)"=w708) -> ("report out"=w711:refnum<class "NI_report.lvclass">, "error out"=w712:errorcluster)  [unwired: 8 in, 1 out]
                n344 = call-poly <vilib>:"Word Easy Table.vi"("report in"=w711, "column headers"=string[] ["框号", "长/mm", "宽/mm", "面积/mm2", "Z值/mm", "部位", "类型", "合格性"], "data"=w707, "error in (no error)"=w712) -> ("report out"=w706:refnum<class "NI_report.lvclass">, "error out"=w705:errorcluster)  [unwired: 9 in, 1 out]
              }
              frame #5 {
                n345 = local read "穿透图原始路径"() -> (w720:path)
                n346 = local read "报告模式"() -> (w718:string)
                n347 = Path To String(path=w720) -> (string=w724:string)
                n348 = String Length(string=w724) -> (length=w725:i32)
                n349 = Subtract(x=w725, y=4) -> (x-y=w726:i32)
                n350 = Concatenate Strings("_" ("字符串"), w718, "_.docx" ("字符串")) -> (w716:string)
                n351 = Replace Substring(3:w726, 4:w716, 5:w724) -> (1:w723:string)  [unwired: 1 in, 1 out]
                n352 = String To Path(string=w723) -> (path=w721:path)
                "添加的路径" <- w721
                n353 = call-dynamic "Save Report to File.vi"("report in"=w728, "report file path"=w721, "prompt to replace? (F)"=TRUE, "error in (no error)"=w727) -> ("report out"=w732:refnum<class "NI_report.lvclass">, "error out"=w731:errorcluster)  [unwired: 10 in]
                n354 = call <vilib>:"Word Bring to Front.vi"("report in"=w732, "window state (maximized)"=enum16{"maximized", "minimized", "normal"}."normal", "error in (no error)"=w731) -> ()  [unwired: 11 in, 2 out]
              }
              frame #6 {
                w733 = string[][] [] ("弥散类检测结果合并")
                n355 = local write "弥散类检测结果合并"(w733) -> ()
                n356 = local write "分层类检测结果合并"(w733) -> ()
                n357 = One Button Dialog(message="完成评定并退出程序！\n请查看word报告" ("消息")) -> ()  [unwired: 1 in, 1 out]
              }
            }
          }
        }
      }
      event "stop": Value Change {
        # "退出软件"
        n358 = event-data() -> ("NewVal"=w738:bool)  [unwired: 1 in, 4 out]
        n359 = Two Button Dialog(message="是否关闭本软件？" ("消息")) -> (T button?=w739:bool)  [unwired: 2 in]
        n360 = And(x=w738, y=w739) -> (x .and. y?=w737:bool)
        n361 = case shown="真" w737 {
          frame False {
          }
          frame True {
            w740 = TRUE ("All Images? (No)")
            n362 = local read "穿透图"() -> (w742:T1)
            n363 = local read "反射图"() -> (w741:T1)
            n364 = call "IMAQ Dispose"("All Images? (No)"=w740, "Image"=w742) -> ()  [unwired: 4 in, 1 out]
            n365 = call "IMAQ Dispose"("All Images? (No)"=w740, "Image"=w741) -> ()  [unwired: 4 in, 1 out]
            n366 = disable-structure shown="RUN_TIME_ENGINE==True" {
              frame condition #0 {
                n367 = Quit LabVIEW() -> ()  [unwired: 1 in]
              }
              frame condition #1 (active) {
                n368 = Stop() -> ()  [unwired: 1 in]
              }
            }
          }
        }
      }
    }
  }
  n369 = disable-structure shown="禁用" {
    frame Disabled {
      n370 = while {
        stop <- FALSE stop-if-true
        n371 = local read "查看评定结果"() -> (w745:bool)
        n372 = local read "删除标注"() -> (w746:bool)
        n373 = Or(x=w746, y=w745) -> (x .or. y?=w747:bool)
        n374 = local write "开始标注"(w747) -> ()
        n375 = Wait Until Next ms Multiple(millisecond multiple=u32 50 ("毫秒倍数")) -> ()  [unwired: 1 out]
      }
    }
    frame Enabled {
    }
  }
  "临界面积百分比值" <- w3
  "输入的灰度阈值" <- w4
